vi "Auto InTake.vi"() -> ()   [LabVIEW 2013]
uses:
  Specials/Global Data.vi
panel:
  in  "error in (no error)":errorcluster
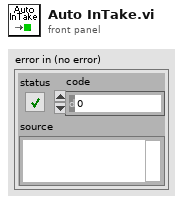
[diagram p1: front panel]
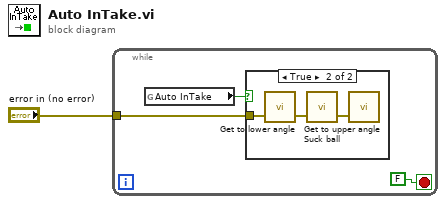
[diagram p0: block diagram]
diagram:
  n1 = while {
    tunnel: "error in (no error)" -> [w4]
    stop <- FALSE stop-if-true
    n2 = global read "Global Data.vi" "Auto InTake"() -> (w2:bool)
    n3 = case shown="True" w2 {
      tunnel: w4 -> [_ w5]
      frame False {
      }
      frame True {
        n4 = call "Get to lower angle.vi"("error in (no error)"=w5) -> ("error out"=w6:errorcluster)  [unwired: 2 in]
        n5 = call "Suck ball.vi"("error in (no error)"=w6) -> ("error out"=w7:errorcluster)  [unwired: 2 in]
        n6 = call "Get to upper angle.vi"("error in (no error)"=w7) -> ()  [unwired: 2 in, 1 out]
      }
    }
  }
